vi "Get Xbox Controller Input.vi"(8 "error in (no error)":errorcluster, 11 "XBox Controller-Virtual in":refnum<class "XBox Controller-Virtual.lvclass">) -> (0 "error out":errorcluster, 3 "XBox Controller-Virtual out":refnum<class "XBox Controller-Virtual.lvclass">)   [LabVIEW 2013, in "XBox Controller.lvlib" / "XBox Controller-Virtual.lvclass"]
uses:
  XBox Controller-Virtual.lvclass
  Robot/Virtual Systems/XBox Controller/XBox Controller Class/XBox Controller-Logical.lvclass
  XBox Controller-Virtual.lvclass/XBox Controller-Virtual.ctl
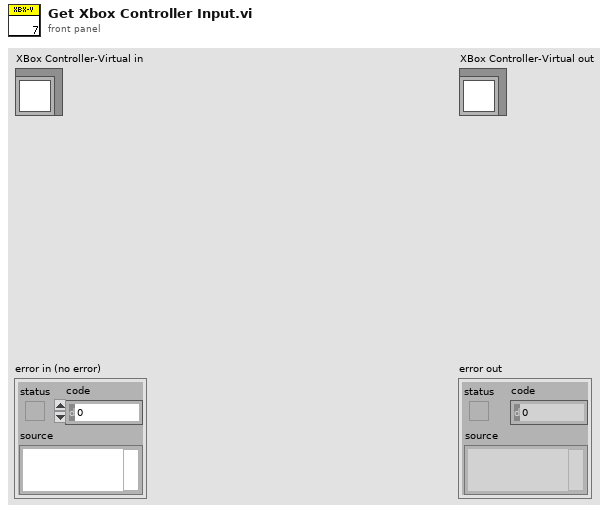
[diagram p1: front panel]
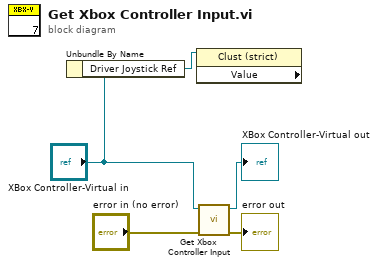
[diagram p0: block diagram]
diagram:
  n1 = Unbundle By Name("XBox Controller-Virtual in") -> ("Driver Joystick Ref"=w1:refnum<vi>)
  n2 = property class="Clust (strict)" props=["Value"](reference=w1) -> ()  [unwired: 1 in, 3 out]
  n3 = call-parent "Get Xbox Controller Input.vi"("error in (no error)"="error in (no error)", "XBox Controller-Logical in"="XBox Controller-Virtual in") -> ("error out"=→"error out":errorcluster, "XBox Controller-Logical out"=→"XBox Controller-Virtual out":refnum<class "XBox Controller-Virtual.lvclass">)  [unwired: 8 in]
